vi "levelChoice.vi"(8 "error in (no error)":errorcluster, 10 "Level Number":u8, 11 "simonMessages in":refnum<class "simonMessages.lvclass">) -> (0 "error out":errorcluster, 3 "simonMessages out":refnum<class "simonMessages.lvclass">)   [LabVIEW 2019, in "simonMessages.lvclass"]
uses:
  simonMessages.lvclass
  simonMessages.lvclass/simonMessages.ctl
  TextDisplay/TextDisplay Class.lvclass
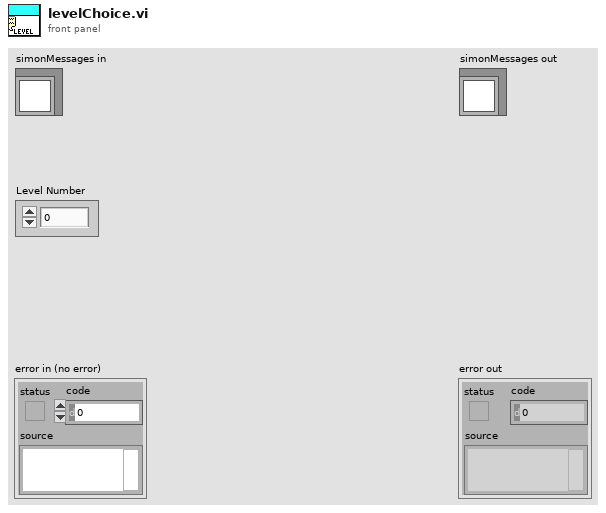
[diagram p1: front panel]
types:
  T1 = cluster{"Text":string, "Size":u8, "Justification":enum16{"Left", "Center", "Right"}, "Display Type":string}
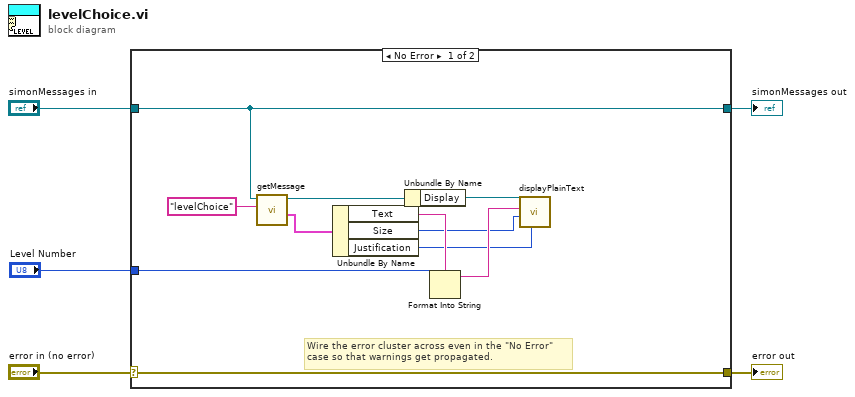
[diagram p0: block diagram]
diagram:
  n1 = case shown="No Error" "error in (no error)" {
    selector: "error in (no error)" -> [w16 w18]
    tunnel: [w16 w18] -> w4
    tunnel: [w10 w17] -> w2
    tunnel: "simonMessages in" -> [w10 w17]
    tunnel: "Level Number" -> [w9 _]
    frame No Error {
      # "Wire the error cluster across even in the \"No Error\"\ncase so that warnings get propagated."
      n2 = call "getMessage.vi"("key"="levelChoice", "simonMessages in"=w10) -> ("Message Cluster"=w12:T1, "simonMessages out"=w15:refnum<class "simonMessages.lvclass">)  [unwired: 7 in, 1 out]
      n3 = Unbundle By Name(w12) -> ("Text"=w8:string, "Size"=w7:u8, "Justification"=w6:enum16{"Left", "Center", "Right"})
      n4 = Unbundle By Name(w15) -> ("Display"=w13:refnum<class "TextDisplay Class.lvclass">)
      n5 = Format Into String(format string=w8, w9) -> (resulting string=w11:string)  [unwired: 2 in, 1 out]
      n6 = call "displayPlainText.vi"("Justification"=w6, "Font Size"=w7, "Text In"=w11, "TextDisplay Class in"=w13) -> ()  [unwired: 6 in, 2 out]
    }
    frame Error {
    }
  }
  "error out" <- w4
  "simonMessages out" <- w2
